vi "matrix pgm.vi"(6 "matrixSize":i32, 7 "normalize":i32, 9 "gamma":i32, 10 "matrix in 2D":dbl[][](array[numeric]), 11 "Path In":path) -> (3 "matrix out 2D":dbl[][](array[numeric]))   [LabVIEW 2012, in "LightPipes.lvlib"]
doc: "__declspec(dllexport) void matrix_pgm(const char *path, double matrix[], int gamma, int normalize, int matrixSize);"
uses:
  LightPipes.lvlib
  Lightpipes.dll
panel:
  out "error out":errorcluster
  in  "n_grid":i32
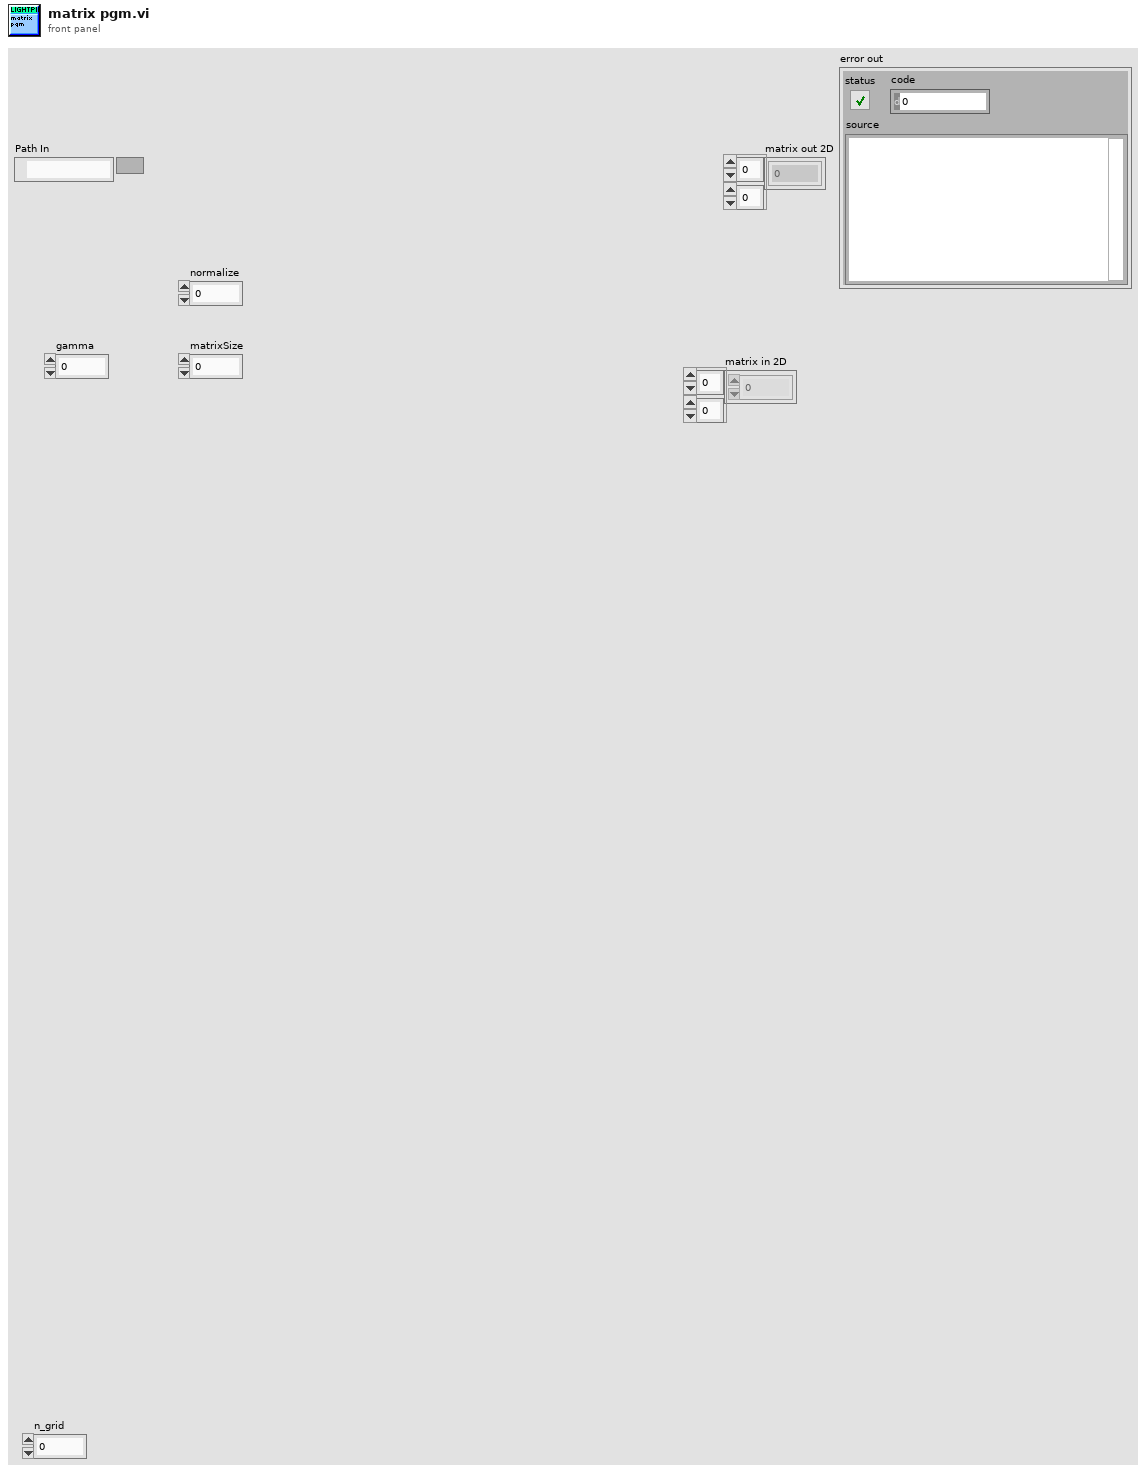
[diagram p1: front panel]
types:
  T1 = enum16{"open", "replace", "create", "open or create", "replace or create", "replace or create with confirmation"}
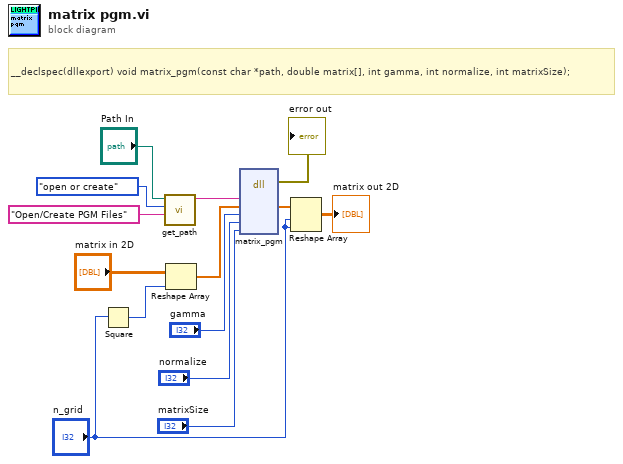
[diagram p0: block diagram]
diagram:
  # "__declspec(dllexport) void matrix_pgm(const char *path, double matrix[], int gamma, int normalize, int matrixSize);"
  n1 = Square(x="n_grid") -> (x^2=w10:i32)
  n2 = call "get_path.vi"("Message Prompt"="Open/Create PGM Files", "operation (default: open/create)"=T1."open or create", "Path In"="Path In") -> ("Path out"=w5:string)  [unwired: 8 in]
  n3 = Reshape Array("matrix in 2D", w10) -> (w9:dbl[])
  n4 = dll-call lib="C:/Users/Tri/Documents/Gerchberg/Lightpipes.*" fn="matrix_pgm"("path"=w5, "matrix"=w9, "gamma"="gamma", "normalize"="normalize", "matrixSize"="matrixSize") -> (error out=→"error out":errorcluster, "matrix"=w8:dbl[])  [unwired: 8 in, 1 out]
  n5 = Reshape Array(w8, "n_grid", "n_grid") -> (→"matrix out 2D":dbl[][])
